vi "CTIOTF_FGV.vi"(8 "error in":errorcluster, 10 "Set_Get":enum16{"Set", "Get"}(ring), 11 "aotfset":bool=TRUE) -> (0 "error out":errorcluster, 3 "aotfGet":bool)   [LabVIEW 2010]
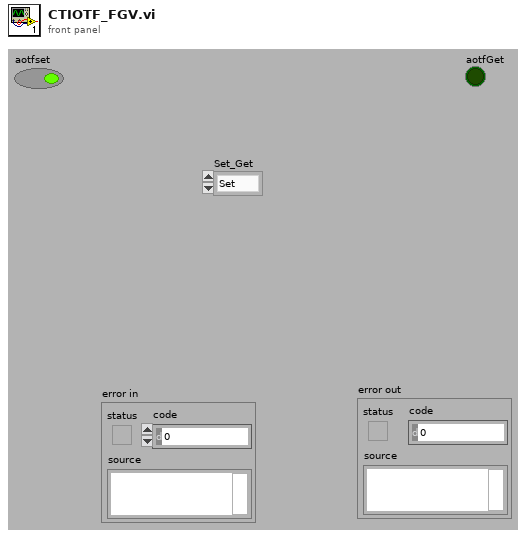
[diagram p1: front panel]
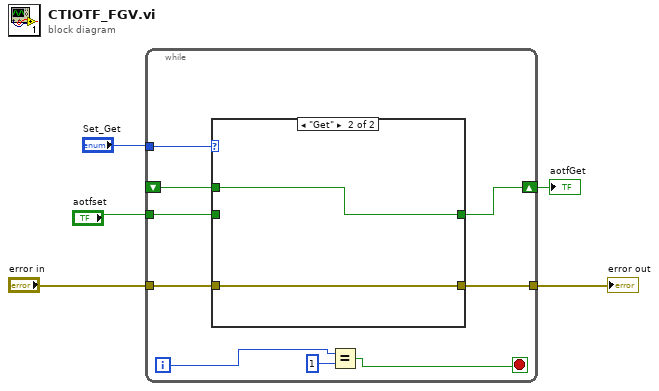
[diagram p0: block diagram]
diagram:
  n1 = while {
    tunnel: "Set_Get" -> [w14]
    tunnel: "aotfset" -> [w13]
    shift-right: [w12] -> w3
    shift-left: _ -> [w11]
    tunnel: "error in" -> [w7]
    tunnel: [w6] -> w1
    i -> [w8]
    stop <- w9 stop-if-true
    n2 = case shown="\"Get\"" w14 {
      tunnel: w13 -> [w16 _]
      tunnel: [w16 w18] -> w12
      tunnel: w11 -> [_ w18]
      tunnel: w7 -> [w15 w17]
      tunnel: [w15 w17] -> w6
      frame "Set", Default {
      }
      frame "Get" {
      }
    }
    n3 = Equal?(x=w8, y=1) -> (x = y?=w9:bool)
  }
  "aotfGet" <- w3
  "error out" <- w1
